vi "Make Setup Error Case.vi"(8 "error in (no error)":errorcluster, 11 "Error Checking Test in":refnum<class "Error Checking Test.lvclass">) -> (0 "error out":errorcluster, 3 "LUnit Test Case V2 out":refnum<class "LUnit Test Case V2.lvclass">)   [LabVIEW 2020, in "Error Checking Test.lvclass"]
uses:
  Error Checking Test.lvclass
  LUnit Test Case/LUnit Test Case V2.lvclass
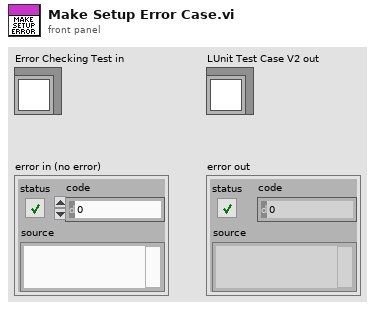
[diagram p1: front panel]
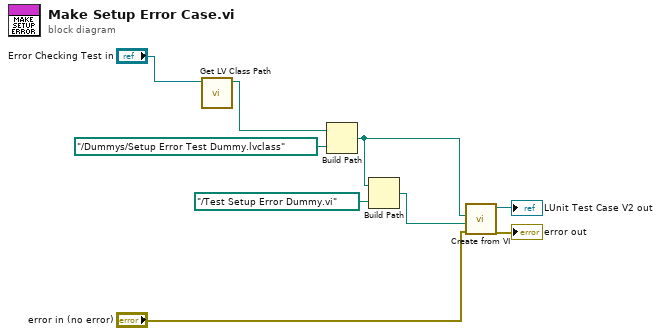
[diagram p0: block diagram]
diagram:
  n1 = call <vilib>:"Get LV Class Path.vi"("object"="Error Checking Test in") -> ("class path"=w2:path)  [unwired: 9 in, 1 out]
  n2 = Build Path(base path=w2, name or relative path=path "../Dummys/Setup Error Test Dummy.lvclass") -> (appended path=w4:path)
  n3 = Build Path(base path=w4, name or relative path=path "../Test Setup Error Dummy.vi") -> (appended path=w6:path)
  n4 = call "Create from VI.vi"("error in (no error)"="error in (no error)", "Test Method VI Path"=w6, "Test Case LVCLass Path"=w4) -> ("error out"=→"error out":errorcluster, "LUnit Test Case V2 out"=→"LUnit Test Case V2 out":refnum<class "LUnit Test Case V2.lvclass">)  [unwired: 7 in]
